vi "Teleop.vi"(10 "Match Info":T1={"Autonomous Elapsed Seconds"=0.0, "TeleOp Elapsed Seconds"=0.0, "Disabled Elapsed Seconds"=0.0, "Visited Autonomous"=FALSE, "Visited TeleOp"=FALSE, "Visited Disabled"=FALSE, "Autonomous Settings"={"Autonomous Style"=enum."Independent", "VI Refnum"=refnum}}, 11 "Call Context":T2) -> ()   [LabVIEW 2014]
doc: "This VI is called for each TeleOp packet received from the DS where the robot is not disabled. It is often used to read from the joysticks and update I/O or to update setpoints for timed control loops. It should complete and return within 20 milliseconds or it may miss DS packets."
uses:
  <vilib>/Rock Robotics/WPI/DriverStation/WPI_DriverStationDerivedRobotMode.ctl
  <vilib>/Rock Robotics/WPI/DriverStation/WPI_DriverStationMatch Info.ctl
  <vilib>/Rock Robotics/WPI/Solenoid/WPI_SolenoidValue.ctl
  Global Variables.vi
  <vilib>/Rock Robotics/WPI/Joystick/WPI_JoystickGetSetRefNum.vi
  <vilib>/Rock Robotics/WPI/Solenoid/WPI_SolenoidSetEnum.vi
panel:
  in  "Deploy?":bool
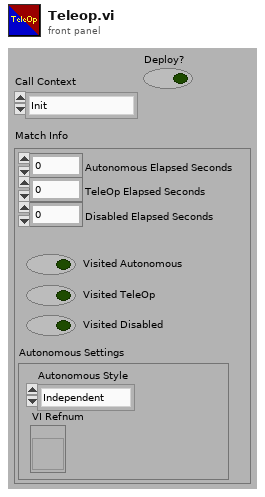
[diagram p1: front panel]
types:
  T1 = typedef "WPI_DriverStationMatch Info.ctl" = cluster{"Autonomous Elapsed Seconds":dbl, "TeleOp Elapsed Seconds":dbl, "Disabled Elapsed Seconds":dbl, "Visited Autonomous":bool, "Visited TeleOp":bool, "Visited Disabled":bool, "Autonomous Settings":cluster{"Autonomous Style":enum16{"Iterative", "Independent"}, "VI Refnum":refnum<vi>}}
  T2 = typedef "WPI_DriverStationDerivedRobotMode.ctl" = enum16{"Init", "Execute", "Stop"}
  T3 = typedef "WPI_SolenoidValue.ctl" = enum16{"Off", "On", "Forward", "Reverse"}
  T4 = typedef "WPI_JoystickDevRef.ctl" = cluster{"Device":T5}
  T5 = typedef "WPI_JoystickDeviceEnum.ctl" = enum16{"USB 0", "USB 1", "USB 2", "USB 3", "USB 4", "USB 5"}
  T6 = typedef "WPI_SolenoidDevRef.ctl" = cluster{"DevStatus":errorcluster, "Pneumatics Control Module":u8, "Forward Solenoid Channel":T7, "Reverse Solenoid Channel":T7}
  T7 = typedef "WPI_SolenoidChannel.ctl" = enum8{"Solenoid 0", "Solenoid 1", "Solenoid 2", "Solenoid 3", "Solenoid 4", "Solenoid 5", "Solenoid 6", "Solenoid 7", "Invalid"}
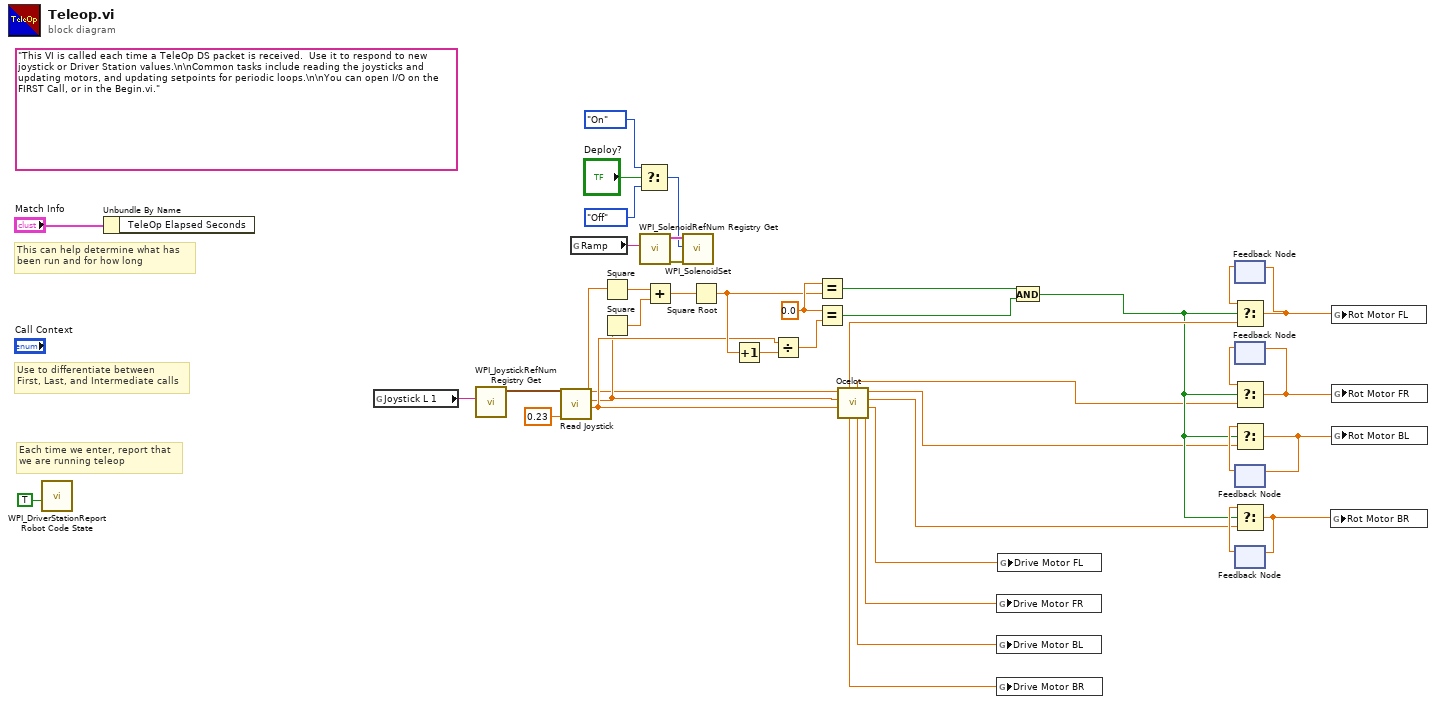
[diagram p0: block diagram]
diagram:
  w33 = 0.0 ("x")
  (unwired) "This VI is called each time a TeleOp DS packet is received.  Use it to respond to new joystick or Driver Station values.\n\nCommon tasks include reading the joysticks and updating motors, and updating setpoints for periodic loops.\n\nYou can open I/O on the FIRST Call, or in the Begin.vi."
  # "Each time we enter, report that\nwe are running teleop"
  # "Use to differentiate between\nFirst, Last, and Intermediate calls"
  # "This can help determine what has\nbeen run and for how long"
  n1 = call <vilib>:"WPI_DriverStationReport Robot Code State.vi"("TeleOp"=TRUE ("Autonomous")) -> ()  [unwired: 10 in, 1 out]
  n2 = Unbundle By Name("Match Info") -> ()  [unwired: 1 out]
  n3 = global read "Global Variables.vi" "Joystick L 1"() -> (w39:string)
  n4 = call <vilib>:"WPI_JoystickRefNum Registry Get.vi"("refnum name"=w39) -> ("JoystickDevRef"=w38:T4)  [unwired: 1 in, 9 out]
  n5 = call "Read Joystick.vi"("Joystick Deadbanded Value (default of 0.1)"=0.23, "Joystick L 1 DevRef"=w38) -> ("Joystick R 2 X Axis"=w29:dbl, "Joystick L 1 Y Axis"=w28:dbl, "Joystick L 1 X Axis"=w27:dbl)  [unwired: 7 in]
  n6 = global read "Global Variables.vi" "Ramp"() -> (w5:string)
  n7 = Square(x=w27) -> (x^2=w35:dbl)
  n8 = Square(x=w28) -> (x^2=w36:dbl)
  n9 = Select(t=WPI_SolenoidValue."On" ("Value"), s="Deploy?", f=WPI_SolenoidValue."Off" ("Value")) -> (s? t:f=w2:T3)
  n10 = call <vilib>:"WPI_SolenoidRefNum Registry Get.vi"("refnum name"=w5) -> ("error out"=w6:errorcluster, "SolenoidDevRef"=w7:T6)  [unwired: 9 in]
  n11 = Add(x=w35, y=w36) -> (x+y=w34:dbl)
  n12 = call-poly <vilib>:"WPI_SolenoidSet.vi"("error in (no error)"=w6, "Value"=w2, "SolenoidDevRef"=w7) -> ()  [unwired: 7 in, 2 out]
  n13 = Square Root(x=w34) -> (sqrt(x)=w32:dbl)
  n14 = Increment(x=w32) -> (x+1=w31:dbl)
  n15 = Divide(x=w29, y=w31) -> (x/y=w30:dbl)
  n16 = Equal?(x=w33, y=w32) -> (x = y?=w21:bool)
  n17 = Equal?(x=w33, y=w30) -> (x = y?=w20:bool)
  n18 = call "Ocelot.vi"("RCW (X2)"=w29, "FWD (Y)"=w28, "STR (X)"=w27) -> ("FRD"=w10:dbl, "FLD"=w11:dbl, "BRS"=w12:dbl, "BLS"=w13:dbl, "BLD"=w9:dbl, "FRS"=w14:dbl, "BRD"=w8:dbl, "FLS"=w22:dbl)  [unwired: 1 in]
  n19 = global write "Global Variables.vi" "Drive Motor FR"(w10) -> ()
  n20 = global write "Global Variables.vi" "Drive Motor BL"(w9) -> ()
  n21 = global write "Global Variables.vi" "Drive Motor BR"(w8) -> ()
  n22 = global write "Global Variables.vi" "Drive Motor FL"(w11) -> ()
  n23 = And(x=w21, y=w20) -> (x .and. y?=w19:bool)
  n24 = feedback #1() -> (w26:dbl)  [unwired: 1 in]
  n25 = Select(t=w26, s=w19, f=w22) -> (s? t:f=w18:dbl)
  n26 = feedback-in #1(w18) -> ()
  n27 = feedback #2() -> (w25:dbl)  [unwired: 1 in]
  n28 = Select(t=w25, s=w19, f=w14) -> (s? t:f=w17:dbl)
  n29 = feedback-in #2(w17) -> ()
  n30 = feedback #3() -> (w24:dbl)  [unwired: 1 in]
  n31 = Select(t=w24, s=w19, f=w13) -> (s? t:f=w16:dbl)
  n32 = feedback-in #3(w16) -> ()
  n33 = feedback #4() -> (w23:dbl)  [unwired: 1 in]
  n34 = Select(t=w23, s=w19, f=w12) -> (s? t:f=w15:dbl)
  n35 = feedback-in #4(w15) -> ()
  n36 = global write "Global Variables.vi" "Rot Motor BR"(w15) -> ()
  n37 = global write "Global Variables.vi" "Rot Motor FL"(w18) -> ()
  n38 = global write "Global Variables.vi" "Rot Motor FR"(w17) -> ()
  n39 = global write "Global Variables.vi" "Rot Motor BL"(w16) -> ()
